vi "PAN_ExpScript.vi"(7 "macrodir":path, 8 "error in (no error)":errorcluster, 10 "script":string) -> (0 "error out":errorcluster)   [LabVIEW 2016]
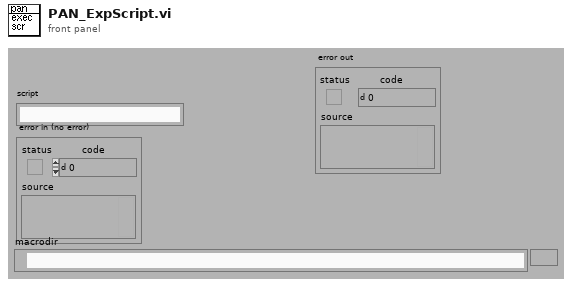
[diagram p1: front panel]
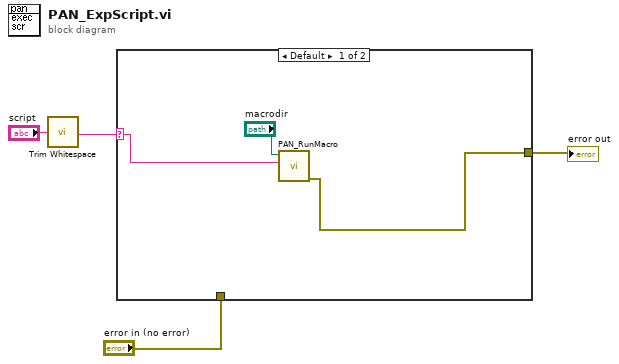
[diagram p0: block diagram]
diagram:
  n1 = call <vilib>:"Trim Whitespace.vi"("string"="script") -> ("trimmed string"=w1:string)  [unwired: 1 in]
  n2 = case shown="Default" w1 {
    selector: w1 -> [w6 _]
    tunnel: [w7 w8] -> w3
    tunnel: "error in (no error)" -> [_ w8]
    frame Default {
      n3 = call "PAN_RunMacro.vi"("commands"=w6, "macrodir"="macrodir") -> ("error out"=w7:errorcluster)  [unwired: 1 in, 8 out]
    }
    frame "", "none" {
    }
  }
  "error out" <- w3
